vi "niRFUtil WFM Remove Origin Offset - Mean Average.vi"(0 "Signal In":T1 {"y" format="%.2f"; "dx" format="%^.2e"; "x0" format="%^.2e"}) -> (4 "Signal Out":T1 {"y" format="%.2f"; "dx" format="%^.2e"; "x0" format="%^.2e"}, 13 "Origin Offset, dBc":sgl format="%.2f", 14 "Origin Offset":csg format="%.3f")   [LabVIEW 2015, in "niRFUtil.lvlib"]
doc: "(c) Copyright 2006, National Instruments, Inc. This VI may not be duplicated, sold, or distributed without written consent from National Instruments."
uses:
  niRFUtil.lvlib
  Includes/niRFUtil INC Complex Waveform.ctl
  Includes/niRFUtil INC Complex Array.ctl
  Measurements/niRFUtil MEAS Mean (complex array).vi
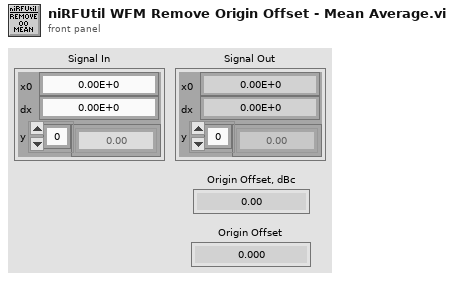
[diagram p1: front panel]
types:
  T1 = typedef "niRFUtil.lvlib/niRFUtil INC Complex Waveform.ctl" = cluster{"x0":dbl, "dx":dbl, "y":T2}
  T2 = typedef "niRFUtil.lvlib/niRFUtil INC Complex Array.ctl" = csg[]
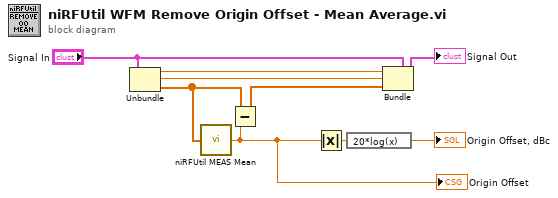
[diagram p0: block diagram]
diagram:
  n1 = Unbundle("Signal In") -> ("x0"=w6:dbl, "dx"=w5:dbl, "y"=w3:T2)
  n2 = call-poly "niRFUtil MEAS Mean.vi"("Complex Array"=w3) -> ("Mean"=w2:csg)  [unwired: 14 out]
  "Origin Offset" <- w2
  n3 = Subtract(x=w3, y=w2) -> (x-y=w1:T2)
  n4 = Absolute Value(x=w2) -> (abs(x)=w8:sgl)
  n5 = expression code="20*log(x)"(w8) -> (→"Origin Offset, dBc":sgl)
  n6 = Bundle(cluster="Signal In", "x0"=w6, "dx"=w5, "y"=w1) -> (→"Signal Out":T1)
